vi "GetOperationCycleEndTime.vi"(8 "error in":errorcluster, 11 "OperationCycle in":refnum<class "OperationCycle.lvclass">) -> (0 "error out":errorcluster, 2 "OperationRunEndTime":timestamp, 3 "OperationCycle out":refnum<class "OperationCycle.lvclass">)   [LabVIEW 2021, in "ProligentXMLGenerator.lvlib" / "OperationCycle.lvclass"]
doc: "Defines the end date of the operation cycle, i.e. when the unit was routed out of the operation. If 'OperationCycleStatus' is equal to 'NOT_COMPLETED' this value must be ommited. This value must be greater or equal than OperationCycleEndTime.\n\nNote that the if the Data Warehouse already contains this operation cycle but it is not already closed, the OperationCycleEndTime written in the Data Warehouse will be set according to the following rule: OperationCycleEndTime(in database) = OperationCycleStartTime(in database) + (OperationCycleEndTime(from xml) - OperationCycleStartTime(from xml)).\n\nThis attribute cannot be updated.\nThis value is restricted to \"1900-01-01T00:00:00Z\" -\"2100-01-01T00:00:00Z\"."
uses:
  OperationCycle.lvclass
  OperationCycle.lvclass/OperationCycle.ctl
  Base/DateTime/DateTime.lvclass
  Base/Attribute/Attribute.lvclass
  C:/Projects/proligent-xml-generator-labview/src/ProligentXMLGenerator/Base/Attribute/Attribute.lvclass
  C:/Projects/proligent-xml-generator-labview/src/ProligentXMLGenerator/Base/DateTime/DateTime.lvclass
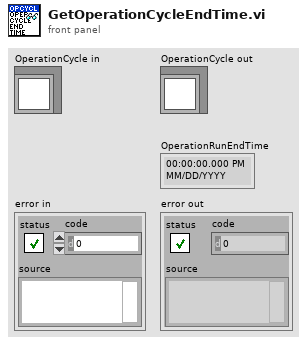
[diagram p1: front panel]
types:
  T1 = typedef "ProligentXMLGenerator.lvlib/OperationCycle.lvclass/Data.ctl" = cluster{"Name":string, "CustomData":refnum<class "CustomData.lvclass">, "ProcessFullName":refnum<class "ProcessFullName.lvclass">, "ProcessVersion":refnum<class "NonEmptyString_64.lvclass">, "OperationCycleId":refnum<class "Guid.lvclass">, "OperationName":refnum<class "NonEmptyString_65.lvclass">, "Location":refnum<class "FullName.lvclass">, "User":refnum<class "NonEmptyString_255.lvclass">, "OperationCycleStatus":refnum<class "ExecutionStatus.lvclass">, "OperationCycleStartTime":refnum<class "DateTime.lvclass">, "OperationCycleEndTime":refnum<class "DateTime.lvclass">, "TimeZoneInfoId":string}
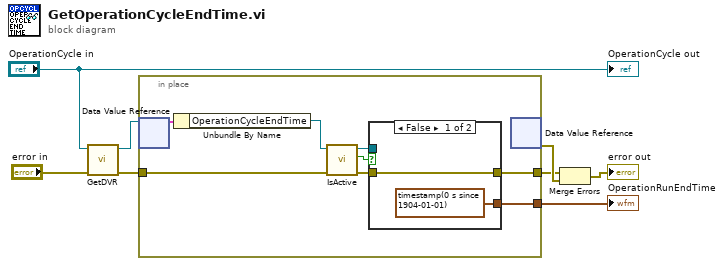
[diagram p0: block diagram]
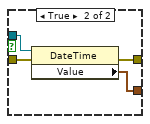
[diagram p2: hidden frame]
diagram:
  n1 = call "GetDVR.vi"("error in"="error in", "OperationCycle in"="OperationCycle in") -> ("error out"=w2:errorcluster, "DVRReference"=w7:refnum<data-value>)  [unwired: 8 in]
  n2 = in-place "In Place Element Structure" {
    in-place-border: [w15] -> w6
    in-place-border: w2 -> [w11]
    in-place-border: [w14] -> w1
    n3 = in-place-dvr #1(w7) -> (w16:T1)  [unwired: 1 out]
    n4 = Unbundle By Name(w16) -> ("OperationCycleEndTime"=w13:refnum<class "DateTime.lvclass">)
    n5 = call "IsActive.vi"("error in"=w11, "Attribute in"=w13) -> ("error out"=w10:errorcluster, "IsActive"=w9:bool, "Attribute in"=w12:refnum<class "DateTime.lvclass">)  [unwired: 7 in]
    n6 = case shown="False" w9 {
      tunnel: [timestamp(0 s since 1904-01-01) ("Value") w22] -> w15
      tunnel: [w17 w21] -> w14
      tunnel: w12 -> [_ w20]
      tunnel: w10 -> [w17 w19]
      frame False {
      }
      frame True {
        n7 = property on="Property Node" class="DateTime"(reference=w20, error in=w19) -> (error out=w21:errorcluster, "Value"=w22:timestamp)  [unwired: 1 out]
      }
    }
    n8 = in-place-dvr #1() -> (w8:errorcluster)  [unwired: 1 in, 1 out]
  }
  "OperationRunEndTime" <- w6
  n9 = Merge Errors(w1, w8) -> (→"error out":errorcluster)
  "OperationCycle out" <- "OperationCycle in"
